vi "Take BL Measurement.vi"(8 "Setup filename":string="Wing_Pressure.xls", 9 "Averaging time (min)":dbl, 10 "File":T1, 11 "Filename":path) -> (1 "Uref":dbl format="%#.3f", 2 "U Trav":dbl, 3 "Z":dbl)   [LabVIEW 2021]
uses:
  Anemometry/Anemometry Sub Vis/Controls/Save_Data.ctl
  Camera Server/Camera enum/Camera resolution.ctl
  Anemometry/Anemometry Sub Vis/Controls/Setup.ctl
  Anemometry/Anemometry Sub Vis/Globals/Meas_global.vi
  Anemometry/Anemometry Sub Vis/Globals/Dynamic_call_global.ph.vi
panel:
  out "Density Kg/m^3":dbl format="%#.3f"
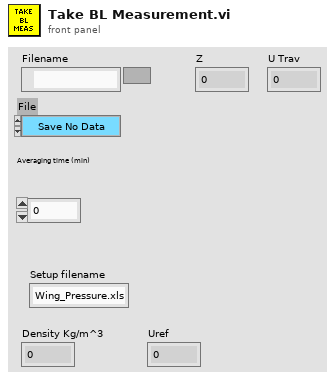
[diagram p1: front panel]
types:
  T1 = typedef "Save_Data.ctl" = enum16{"Save No Data", "Save Data"}
  T2 = typedef "Setup.ctl" = enum16{"Run Program", "Show Setup", "Save Current Setup", "Setup Front Panel"}
  T3 = typedef "Camera resolution.ctl" = u8
  T4 = typedef "Analysis_info_cluster.ctl" = cluster{"Colour":u32, "Inst type":T5, "Inst name":string, "Symbol":string, "Code name":string, "Extra Info":string, "Inst Array":T6, "Extra Titles":string[], "Extra Values":string[], "U":dbl, "u^2":dbl, "u^3":dbl, "u^4":dbl, "Skew_u":dbl, "Kurt_u":dbl, "Sd Error in Mean":dbl, "% u'/U":dbl, "X":dbl, "Y":dbl, "Z":dbl, "Timescale integral Estimate":dbl, "Sd Error in Variance":dbl, "Calib File":path, "Calib Constants":dbl[], "Output Position":bool, "Stats":enum16{"None", "Basic", "Full"}, "Av Sampling Rate":dbl, "Av No of Samples":dbl, "Total Meas Time (s)":dbl, "ADAM Ch Name":string, "Max value":dbl, "Min value":dbl, "Req Sample Rate Hz":dbl, "Sync Delay Time (s)":dbl, "Ch No":i16, "Device":string, "Use Latest Calib":bool, "Port":string, "Metadata Ch Names":string[], "Metadata Ch Values":string[], "Label":string}
  T5 = typedef "Inst_type.ctl" = enum16{"Raw voltage", "Raw with zero offsetting", "Propeller anemometer", "Pressure Transducer", "Pitot-static tube", "Hot wire", "Cross wire 1", "Cross wire 2", "Generic Linear", "Generic Polynomial", "Generic BackPoly", "Fast FID", "Thermocouple", "Cold wire", "Pulsed Wire", "LDA Vel", "LDA Tran time", "LDA Arr time", "Microphone"}
  T6 = typedef "Instrument_Array.ctl" = enum16{"PWA", "LDA", "Analogue"}
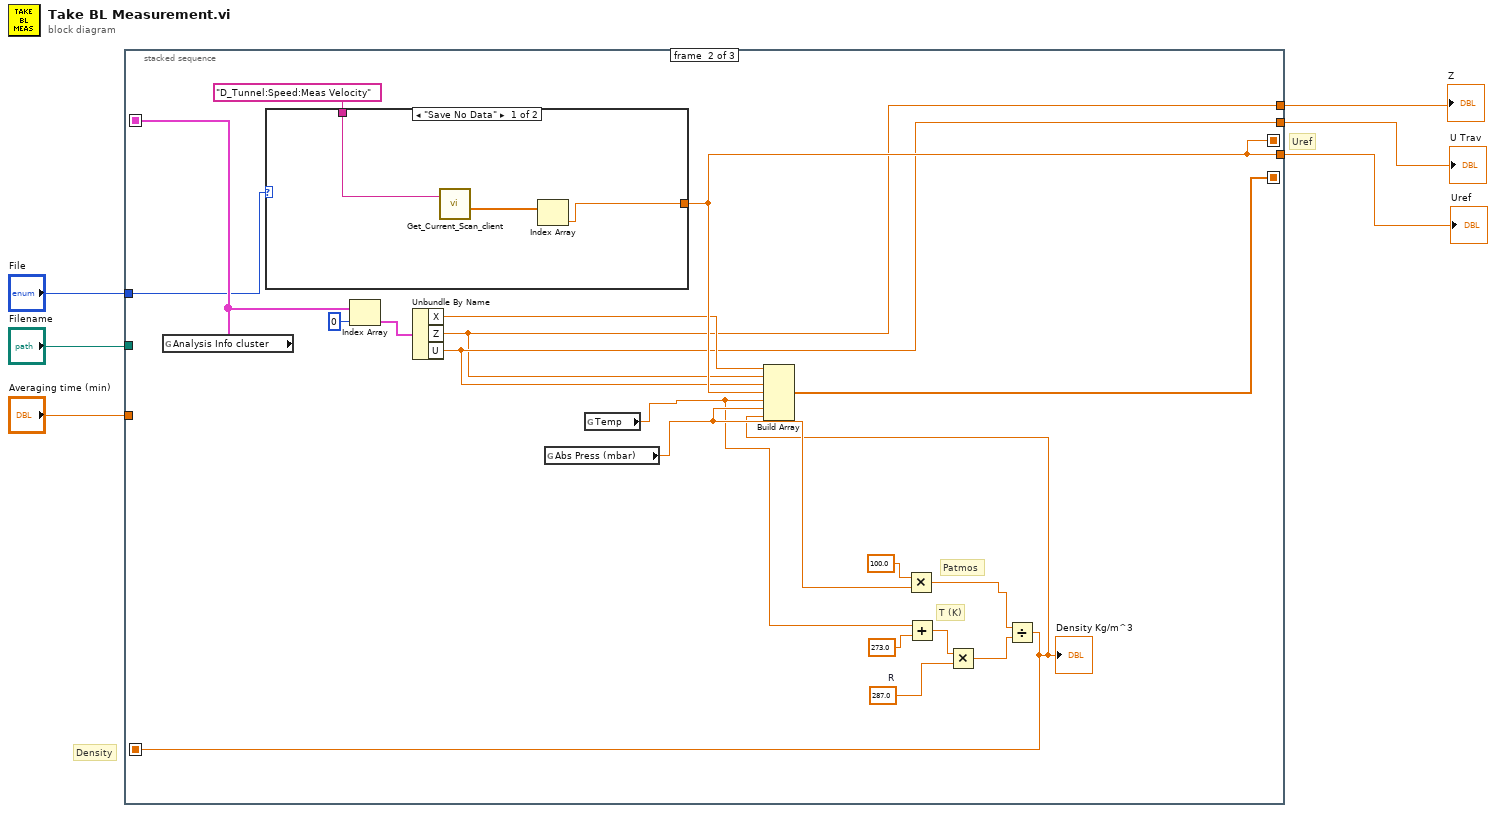
[diagram p0: block diagram]
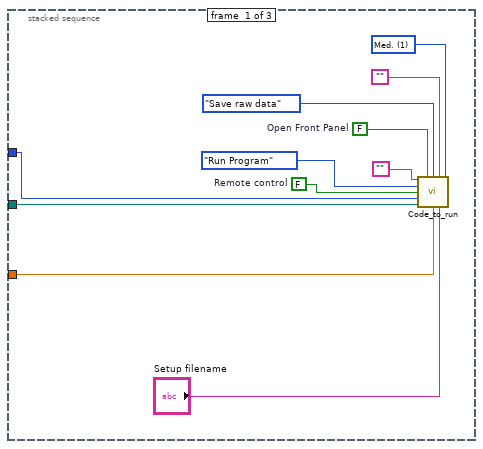
[diagram p2: hidden frame]
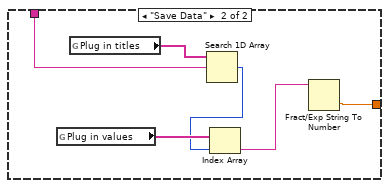
[diagram p3: hidden frame]
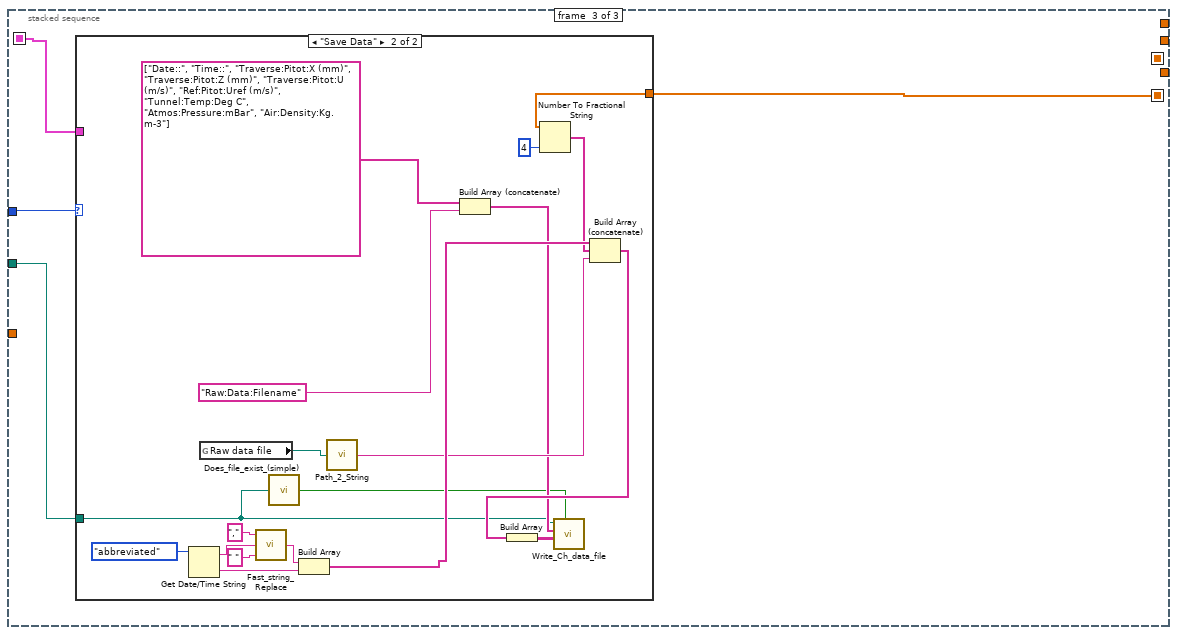
[diagram p4: hidden frame]
diagram:
  # "Uref"
  # "Density"
  n1 = stacked-sequence {
    seq-local: [_ w36 _] -> [_ _ w48]
    seq-local: [_ w35 _] -> [_ _ w47]
    seq-local: [_ w20 _] -> [_ _ _]
    seq-local: [_ w24 _] -> [_ _ _]
    tunnel: "Filename" -> [w10 _ w46]
    tunnel: [_ w24 _] -> w2
    tunnel: [_ w22 _] -> w3
    tunnel: [_ w21 _] -> w4
    tunnel: "Averaging time (min)" -> [w9 _ _]
    tunnel: "File" -> [w8 w19 w49]
    frame #0 {
      w15 = FALSE  # Remote control
      w12 = FALSE  # Open Front Panel
      w17 = T3 1 items=["Low", "Med.", "High", "Max."] ("Camera Resolution")
      n2 = call "Code_to_run.vi"("Extra command String"="", "Open Front Panel"=w12, "Raw data option"=enum16{"Save raw data", "Raw data not saved"}."Save raw data", "Current Row Comments"="", "Camera Resolution"=w17, "setup"=Setup."Run Program", "Remote control"=w15, "File"=w8, "Results Filename"=w10, "Averaging time (min)"=w9, "Setup filename"="Setup filename") -> ()  [unwired: 4 in, 1 out]
    }
    frame #1 {
      w29 = 287.0  # R
      # "T (K)"
      # "Patmos"
      n3 = global read "Meas_global.vi" "Analysis Info cluster"() -> (w36:T4[])
      n4 = case shown="\"Save No Data\"" w19 {
        tunnel: [w37 w41] -> w24
        tunnel: "D_Tunnel:Speed:Meas Velocity" -> [w39 w40]
        frame "Save No Data" {
          n5 = call "Get_Current_Scan_client.vi"("singleChannel"=w39) -> ("Numerical Values"=w38:dbl[])  [unwired: 1 in, 3 out]
          n6 = Index Array(array=w38) -> (element=w37:dbl)  [unwired: 1 in]
        }
        frame "Save Data" {
          n7 = global read "Dynamic_call_global.ph.vi" "Plug in values"() -> (w44:string[])
          n8 = global read "Dynamic_call_global.ph.vi" "Plug in titles"() -> (w45:string[])
          n9 = Search 1D Array(1D array=w45, element=w40) -> (index of element=w43:i32)  [unwired: 1 in]
          n10 = Index Array(array=w44, index=w43) -> (element=w42:string)
          n11 = Fract/Exp String To Number(string=w42) -> (number=w41:dbl)  [unwired: 3 in, 1 out]
        }
      }
      n12 = Index Array(array=w36, index=0) -> (element=w26:T4)
      n13 = Unbundle By Name(w26) -> ("X"=w23:dbl, "Z"=w21:dbl, "U"=w22:dbl)
      n14 = global read "Meas_global.vi" "Abs Press (mbar)"() -> (w34:dbl)
      n15 = global read "Meas_global.vi" "Temp"() -> (w32:dbl)
      n16 = Multiply(x=100.0, y=w34) -> (x*y=w27:dbl)
      n17 = Add(x=w32, y=273.0) -> (x+y=w30:dbl)
      n18 = Multiply(x=w30, y=w29) -> (x*y=w28:dbl)
      n19 = Divide(x=w27, y=w28) -> (x/y=w20:dbl)
      "Density Kg/m^3" <- w20
      n20 = Build Array(w23, w21, w22, w24, w32, w34, w20) -> (w35:dbl[])
    }
    frame #2 {
      n21 = case shown="\"Save Data\"" w49 {
        tunnel: w48 -> [_ _]
        tunnel: w47 -> [_ w50]
        tunnel: w46 -> [_ w52]
        frame "Save No Data", Default {
        }
        frame "Save Data" {
          n22 = Get Date/Time String(date format (0)=enum16{"short", "long", "abbreviated"}."abbreviated") -> (date string=w66:string, time string=w61:string)  [unwired: 2 out]
          n23 = global read "Meas_global.vi" "Raw data file"() -> (w57:path)
          n24 = call "Fast_string_Replace.vi"("Replace match with:"=" ", "Input String"=w66, "regular expression"=",") -> ("Output String"=w62:string)  [unwired: 2 out]
          n25 = call "Does_file_exist_(simple).vi"("Pathname"=w52) -> ("exists?"=w51:bool)
          n26 = Build Array(w62, w61) -> (w59:string[])
          n27 = call "Path_2_String.vi"("Real Path"=w57) -> ("Path String"=w56:string)
          n28 = Build Array (concatenate)(string[] ["Date::", "Time::", "Traverse:Pitot:X (mm)", "Traverse:Pitot:Z (mm)", "Traverse:Pitot:U (m/s)", "Ref:Pitot:Uref (m/s)", "Tunnel:Temp:Deg C", "Atmos:Pressure:mBar", "Air:Density:Kg.m-3"], "Raw:Data:Filename") -> (w53:string[])
          n29 = Number To Fractional String(number=w50, precision (6)=i16 4) -> (F-format string=w58:string[])  [unwired: 2 in]
          n30 = Build Array (concatenate)(w59, w58, w56) -> (w55:string[])
          n31 = Build Array(w55) -> (w54:string[][])
          n32 = call "Write_Ch_data_file.vi"("exists?"=w51, "Channel Values"=w54, "Channel names"=w53, "Filename"=w52) -> ()  [unwired: 4 in, 4 out]
        }
      }
    }
  }
  "Z" <- w4
  "U Trav" <- w3
  "Uref" <- w2
